vi "Merge.vi"(8 "error in (no error)":errorcluster, 9 "Target":string, 10 "Git Implementation":refnum<class "Git Implementation.lvclass">, 11 "Git-Merger in":refnum<class "No-Conflicts Merge.lvclass">) -> (0 "error out":errorcluster, 2 "Status Message":string)   [LabVIEW 2017, in "Git-LabVIEW.lvlib" / "No-Conflicts Merge.lvclass"]
doc: "Perform a merge of the \"Target\" into the current branch. If Target is not specified, then the branch will merge \"the remote-tracking branches that the current branch is configured to use as its upstream\".\nSee https://git-scm.com/docs/git-merge for more details.\nThe Status Message is for display only, and cannot be guaranteed for use with scripting."
uses:
  No-Conflicts Merge.lvclass
  C:/LabVIEW Sources/GitImplementation/Merge Operations/Interface/Merge-Delegate.lvclass
  Implementation/Git Implementation.lvclass
  Interface/CMD Return.ctl
  No-Conflicts Merge.lvclass/No-Conflicts Merge.ctl
  <vilib>/Utility/error.llb/Error Cluster From Error Code.vi
  <vilib>/ErrorRing/Error Ring.xnode
  Interface/Merge-Delegate.lvclass
panel:
  out "CMD Return":T1
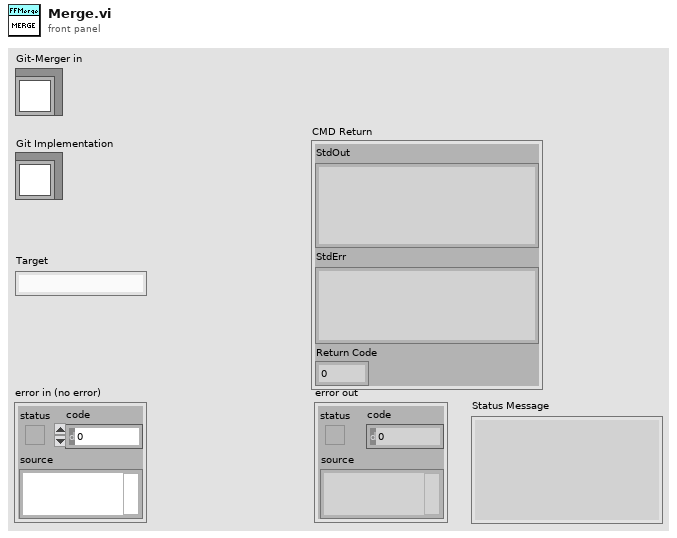
[diagram p1: front panel]
types:
  T1 = typedef "Git-LabVIEW.lvlib/Merge-Delegate.lvclass/CMD Return.ctl" = cluster{"StdOut":string, "StdErr":string, "Return Code":i32}
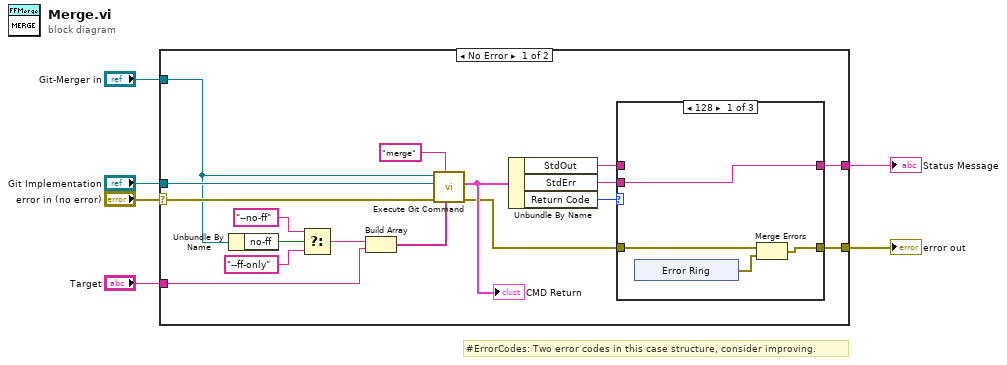
[diagram p0: block diagram]
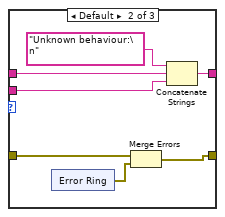
[diagram p2: hidden frame]
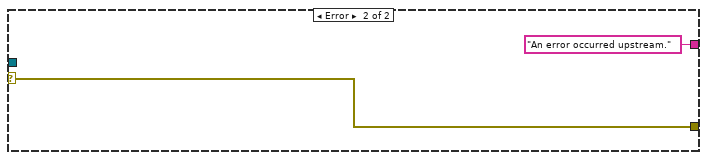
[diagram p4: hidden frame]
diagram:
  # "#ErrorCodes: Two error codes in this case structure, consider improving."
  n1 = case shown="No Error" "error in (no error)" {
    selector: "error in (no error)" -> [w23 w46]
    tunnel: [w11 w46] -> w5
    tunnel: "Git Implementation" -> [w22 _]
    tunnel: "Git-Merger in" -> [w21 _]
    tunnel: "Target" -> [w19 _]
    tunnel: [w10 "An error occurred upstream." ("StdOut")] -> w1
    frame No Error {
      n2 = Unbundle By Name(w21) -> ("no-ff"=w20:bool)
      n3 = Select(t="--no-ff", s=w20, f="--ff-only") -> (s? t:f=w18:string)
      n4 = Build Array(w18, w19) -> (w15:string[])
      n5 = call "Execute Git Command.vi"("Arguments"=w15, "Command"="merge", "error in (no error)"=w23, "Git Implementation"=w22, "Git-Merger in"=w21) -> ("error out"=w7:errorcluster, "CMD Return"=w13:T1)  [unwired: 4 in, 1 out]
      "CMD Return" <- w13
      n6 = Unbundle By Name(w13) -> ("StdOut"=w9:string, "StdErr"=w8:string, "Return Code"=w12:i32)
      n7 = case shown="128" w12 {
        tunnel: w7 -> [w26 w34 w44]
        tunnel: [w24 w33 w44] -> w11
        tunnel: [w27 w37 w43] -> w10
        tunnel: w9 -> [_ w36 w43]
        tunnel: w8 -> [w27 w35 _]
        frame 128 {
          n8 = xnode "Error Ring"() -> ("error out"=w25:errorcluster)
          n9 = Merge Errors(w26, w25) -> (w24:errorcluster)
        }
        frame Default {
          n10 = xnode "Error Ring"() -> ("error out"=w32:errorcluster)
          n11 = Merge Errors(w34, w32) -> (w33:errorcluster)
          n12 = Concatenate Strings("Unknown behaviour:\n" ("StdOut"), w36, w35) -> (w37:string)
        }
        frame 0 {
        }
      }
    }
    frame Error {
    }
  }
  "error out" <- w5
  "Status Message" <- w1
